vi "ED_GetString.vi"(4 "error in":errorcluster, 7 "connection ID in":refnum<k5>) -> (0 "error out":errorcluster, 2 "String":string, 3 "connection ID out":refnum<k5>)   [LabVIEW 2020, in "CAENels EASY-DRIVER.lvlib"]
doc: "When the example is executed, it sets the FAST-PS to CV mode and updates the set-point 10 times per second."
uses:
  CAENels EASY-DRIVER.lvlib
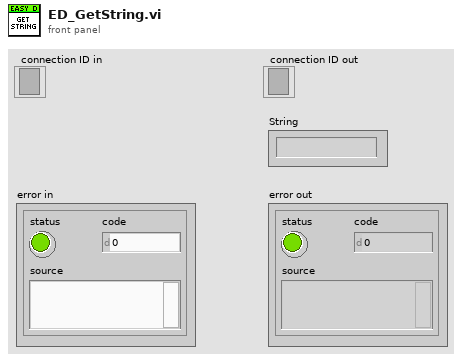
[diagram p1: front panel]
types:
  T1 = enum16{"Standard", "Buffered", "CRLF", "Immediate"}
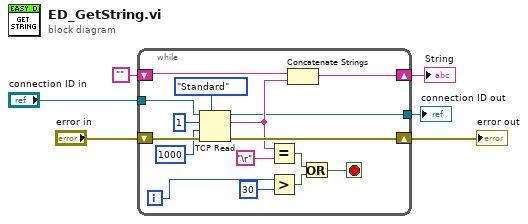
[diagram p0: block diagram]
diagram:
  n1 = while {
    shift-right: [w17] -> w5
    shift-left: "" -> [w19]
    shift-right: [w20] -> w4
    shift-left: "error in" -> [w21]
    tunnel: [w16] -> w3
    tunnel: "connection ID in" -> [w14]
    i -> [w11]
    stop <- w7 stop-if-true
    n2 = TCP Read(connection ID=w14, bytes to read=1, error in (no error)=w21, 7:T1."Standard" ("mode (standard)"), 9:1000 ("timeout ms (25000)")) -> (connection ID out=w16:refnum<k5>, data out=w18:string, error out=w20:errorcluster)
    n3 = Equal?(x=w18, y="\r") -> (x = y?=w8:bool)
    n4 = Greater?(x=w11, y=30) -> (0:w9:bool)
    n5 = Concatenate Strings(w19, w18) -> (w17:string)
    n6 = Or(x=w8, y=w9) -> (x .or. y?=w7:bool)
  }
  "String" <- w5
  "error out" <- w4
  "connection ID out" <- w3
